vi "waveInGetDevCaps.vi"(0 "uDeviceID":u32, 1 "cbwoc":u32=48, 3 "error in (no error)":errorcluster) -> (6 "WaveOutCaps (output)":T1)   [LabVIEW 2012]
uses:
  Windows/System32/winmm.dll
panel:
  out "error out":errorcluster
  out "return type":i32
  in  "WaveOutCaps":T1
  # "waveInGetDevCaps"
  # "typedef struct tagWAVEINCAPSA {\n    WORD    wMid;                    /* manufacturer ID */\n    WORD    wPid;                    /* product ID */\n    MMVERSION vDriverVersion;        /* version of the driver */\n    CHAR    szPname[MAXPNAMELEN];    /* product name (NULL terminated string) */\n    DWORD   dwFormats;               /* formats supported */\n    WORD    wChannels;               /* number of channels supported */\n    WORD    wReserved1;              /* structure packing */\n} WAVEINCAPSA, *PWAVEINCAPSA, *NPWAVEINCAPSA, *LPWAVEINCAPSA;"
  # "typedef unsigned long       DWORD;\ntypedef int                 BOOL;\ntypedef unsigned char       BYTE;\ntypedef unsigned short      WORD;\ntypedef float               FLOAT;\ntypedef FLOAT               *PFLOAT;\ntypedef BOOL near           *PBOOL;\ntypedef BOOL far            *LPBOOL;\ntypedef BYTE near           *PBYTE;\ntypedef BYTE far            *LPBYTE;\ntypedef int near            *PINT;\ntypedef int far             *LPINT;\ntypedef WORD near           *PWORD;\ntypedef WORD far            *LPWORD;\ntypedef long far            *LPLONG;\ntypedef DWORD near          *PDWORD;\ntypedef DWORD far           *LPDWORD;\ntypedef void far            *LPVOID;\ntypedef CONST void far      *LPCVOID;\n\ntypedef int                 INT;\ntypedef unsigned int        UINT;\ntypedef unsigned int        *PUINT;"
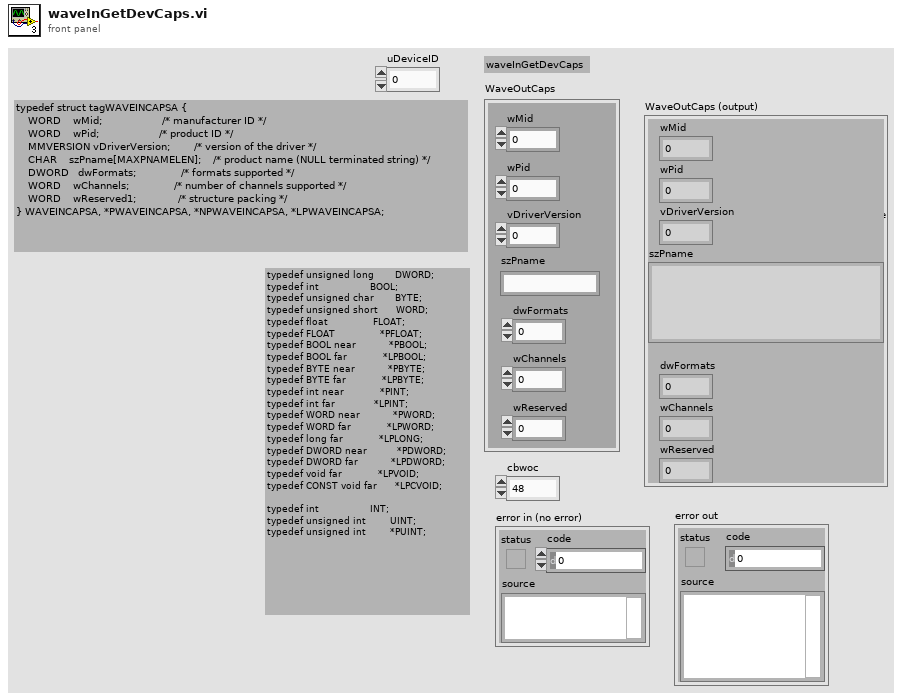
[diagram p1: front panel]
types:
  T1 = cluster{"wMid":u16, "wPid":u16, "vDriverVersion":u32, "szPname":string, "dwFormats":u32, "wChannels":u16, "wReserved":u16}
  T2 = cluster{"U*8 Array[0]":u8, "U*8 Array[1]":u8, "U*8 Array[2]":u8, "U*8 Array[3]":u8, "U*8 Array[4]":u8, "U*8 Array[5]":u8, "U*8 Array[6]":u8, "U*8 Array[7]":u8, "U*8 Array[8]":u8, "U*8 Array[9]":u8, "U*8 Array[10]":u8, "U*8 Array[11]":u8, "U*8 Array[12]":u8, "U*8 Array[13]":u8, "U*8 Array[14]":u8, "U*8 Array[15]":u8, "U*8 Array[16]":u8, "U*8 Array[17]":u8, "U*8 Array[18]":u8, "U*8 Array[19]":u8, "U*8 Array[20]":u8, "U*8 Array[21]":u8, "U*8 Array[22]":u8, "U*8 Array[23]":u8, "U*8 Array[24]":u8, "U*8 Array[25]":u8, "U*8 Array[26]":u8, "U*8 Array[27]":u8, "U*8 Array[28]":u8, "U*8 Array[29]":u8, "U*8 Array[30]":u8, "U*8 Array[31]":u8}
  T3 = cluster{"wMid":u16, "wPid":u16, "vDriverVersion":u32, "U*8 Array":cluster{"U*8 Array[0]":u8, "U*8 Array[1]":u8, "U*8 Array[2]":u8, "U*8 Array[3]":u8, "U*8 Array[4]":u8, "U*8 Array[5]":u8, "U*8 Array[6]":u8, "U*8 Array[7]":u8, "U*8 Array[8]":u8, "U*8 Array[9]":u8, "U*8 Array[10]":u8, "U*8 Array[11]":u8, "U*8 Array[12]":u8, "U*8 Array[13]":u8, "U*8 Array[14]":u8, "U*8 Array[15]":u8, "U*8 Array[16]":u8, "U*8 Array[17]":u8, "U*8 Array[18]":u8, "U*8 Array[19]":u8, "U*8 Array[20]":u8, "U*8 Array[21]":u8, "U*8 Array[22]":u8, "U*8 Array[23]":u8, "U*8 Array[24]":u8, "U*8 Array[25]":u8, "U*8 Array[26]":u8, "U*8 Array[27]":u8, "U*8 Array[28]":u8, "U*8 Array[29]":u8, "U*8 Array[30]":u8, "U*8 Array[31]":u8}, "dwFormats":u32, "wChannels":u16, "wReserved":u16}
  T4 = cluster{"wMid":u16, "wPid":u16, "vDriverVersion":u32, string, "dwFormats":u32, "wChannels":u16, "wReserved":u16}
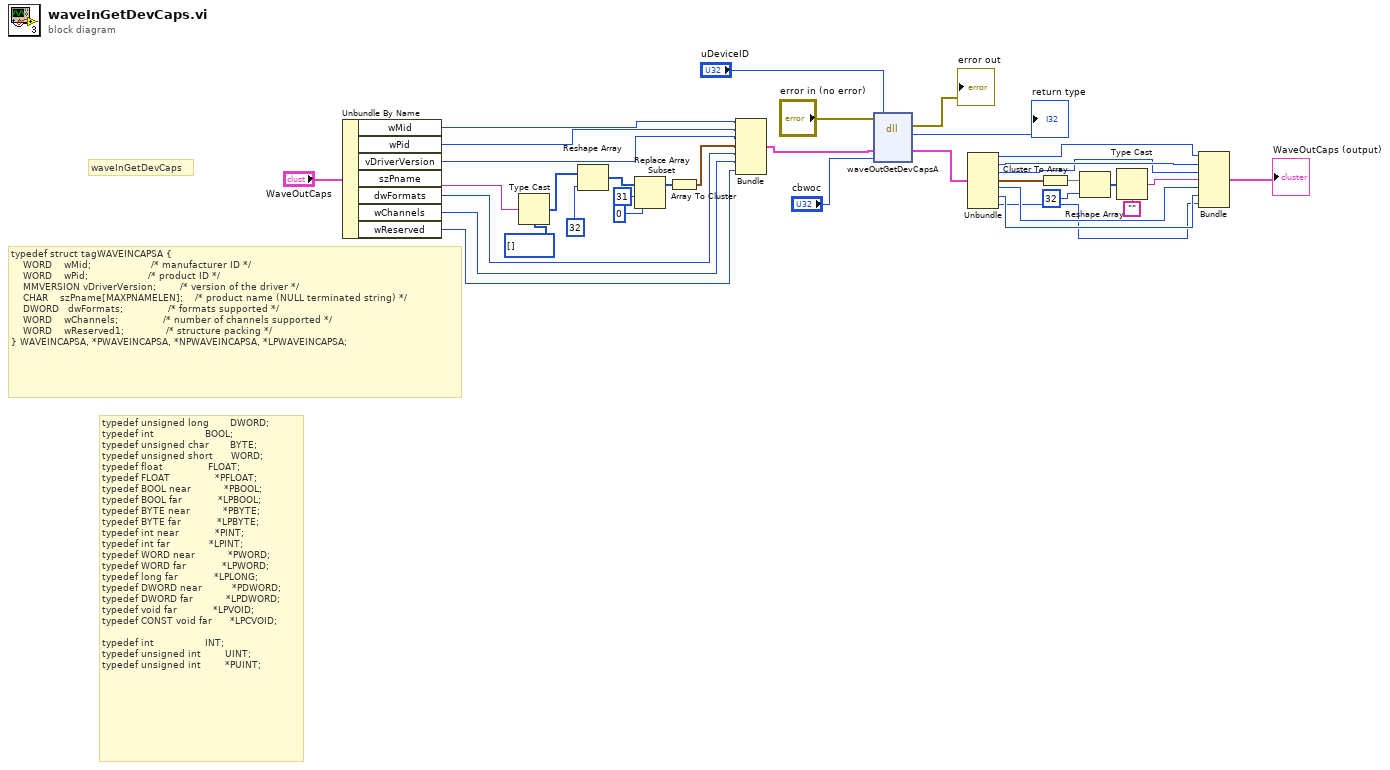
[diagram p0: block diagram]
diagram:
  # "typedef unsigned long       DWORD;\ntypedef int                 BOOL;\ntypedef unsigned char       BYTE;\ntypedef unsigned short      WORD;\ntypedef float               FLOAT;\ntypedef FLOAT               *PFLOAT;\ntypedef BOOL near           *PBOOL;\ntypedef BOOL far            *LPBOOL;\ntypedef BYTE near           *PBYTE;\ntypedef BYTE far            *LPBYTE;\ntypedef int near            *PINT;\ntypedef int far             *LPINT;\ntypedef WORD near           *PWORD;\ntypedef WORD far            *LPWORD;\ntypedef long far            *LPLONG;\ntypedef DWORD near          *PDWORD;\ntypedef DWORD far           *LPDWORD;\ntypedef void far            *LPVOID;\ntypedef CONST void far      *LPCVOID;\n\ntypedef int                 INT;\ntypedef unsigned int        UINT;\ntypedef unsigned int        *PUINT;"
  # "typedef struct tagWAVEINCAPSA {\n    WORD    wMid;                    /* manufacturer ID */\n    WORD    wPid;                    /* product ID */\n    MMVERSION vDriverVersion;        /* version of the driver */\n    CHAR    szPname[MAXPNAMELEN];    /* product name (NULL terminated string) */\n    DWORD   dwFormats;               /* formats supported */\n    WORD    wChannels;               /* number of channels supported */\n    WORD    wReserved1;              /* structure packing */\n} WAVEINCAPSA, *PWAVEINCAPSA, *NPWAVEINCAPSA, *LPWAVEINCAPSA;"
  # "waveInGetDevCaps"
  n1 = Unbundle By Name("WaveOutCaps") -> ("wMid"=w9:u16, "wPid"=w8:u16, "vDriverVersion"=w7:u32, "szPname"=w27:string, "dwFormats"=w5:u32, "wChannels"=w4:u16, "wReserved"=w3:u16)
  n2 = Type Cast(type=u8[] [] ("U*8 Array"), x=w27) -> (*(type *) &x=w28:u8[])
  n3 = Reshape Array(w28, 32 ("dimension size")) -> (w30:u8[])
  n4 = Replace Array Subset(array=w30, new element=u8 0 ("new element/subarray"), index=31) -> (w10:u8[])
  n5 = Array To Cluster(array=w10) -> (cluster=w6:T2)
  n6 = Bundle("wMid"=w9, "wPid"=w8, "vDriverVersion"=w7, "U*8 Array"=w6, "dwFormats"=w5, "wChannels"=w4, "wReserved"=w3) -> (w2:T3)  [unwired: 1 in]
  n7 = dll-call lib="C:/Windows/System32/winmm.dll" fn="waveOutGetDevCapsA"(error in="error in (no error)", "uDeviceID"="uDeviceID", "pwoc"=w2, "cbwoc"="cbwoc") -> (error out=→"error out":errorcluster, "return type"=→"return type":i32, "pwoc"=w23:T3)  [unwired: 4 in, 1 out]
  n8 = Unbundle(w23) -> ("wMid"=w18:u16, "wPid"=w17:u16, "vDriverVersion"=w16:u32, "U*8 Array"=w22:T2, "dwFormats"=w15:u32, "wChannels"=w14:u16, "wReserved"=w13:u16)
  n9 = Cluster To Array(cluster=w22) -> (array=w24:u8[])
  n10 = Reshape Array(w24, 32 ("x")) -> (w21:u8[])
  n11 = Type Cast(type="", x=w21) -> (*(type *) &x=w19:string)
  n12 = Bundle("wMid"=w18, "wPid"=w17, "vDriverVersion"=w16, w19, "dwFormats"=w15, "wChannels"=w14, "wReserved"=w13) -> (→"WaveOutCaps (output)":T4)  [unwired: 1 out]
